vi "写入B版外设配置.vi"(8 "error in (no error)":errorcluster, 10 "外设配置":T1 {"阀型号" items=["垦拓10通阀"]; "总氮x公式0" items=["0", "1"]; "光谱仪类型" items=["1型", "2型", "3型", "2型氙灯联控"]; "泵类型" items=["润泽注射泵", "垦拓注射泵"]}, 11 "MB session in":refnum<class "MB_Master.lvclass">) -> (0 "error out":errorcluster, 3 "MB session out":refnum<class "MB_Master.lvclass">)   [LabVIEW 2016, in "斯坦道总磷总氮.lvlib"]
uses:
  <vilib>/Plasmionique/MB Master/MB_Master/MB_Master.lvclass
  <vilib>/Plasmionique/MB Master/MB_Master_Serial/MB_Master_Serial.lvclass
  C:/Program Files (x86)/National Instruments/LabVIEW 2016/vi.lib/Plasmionique/MB Master/MB_Master/MB_Master.lvclass
  <vilib>/Plasmionique/MB Master/MB Master.lvlib
  <vilib>/Utility/VariantDataType/VariantType.lvlib
panel:
  out "大小":i32
  in  "U32":u32
  in  "SGL":sgl
  in  "U16":u16
  in  "U8":u8
  in  "VISA Resource":refnum<visa-resource-name>
  in  "引用选择":enum16{"MB引用", "自建引用"}(ring)
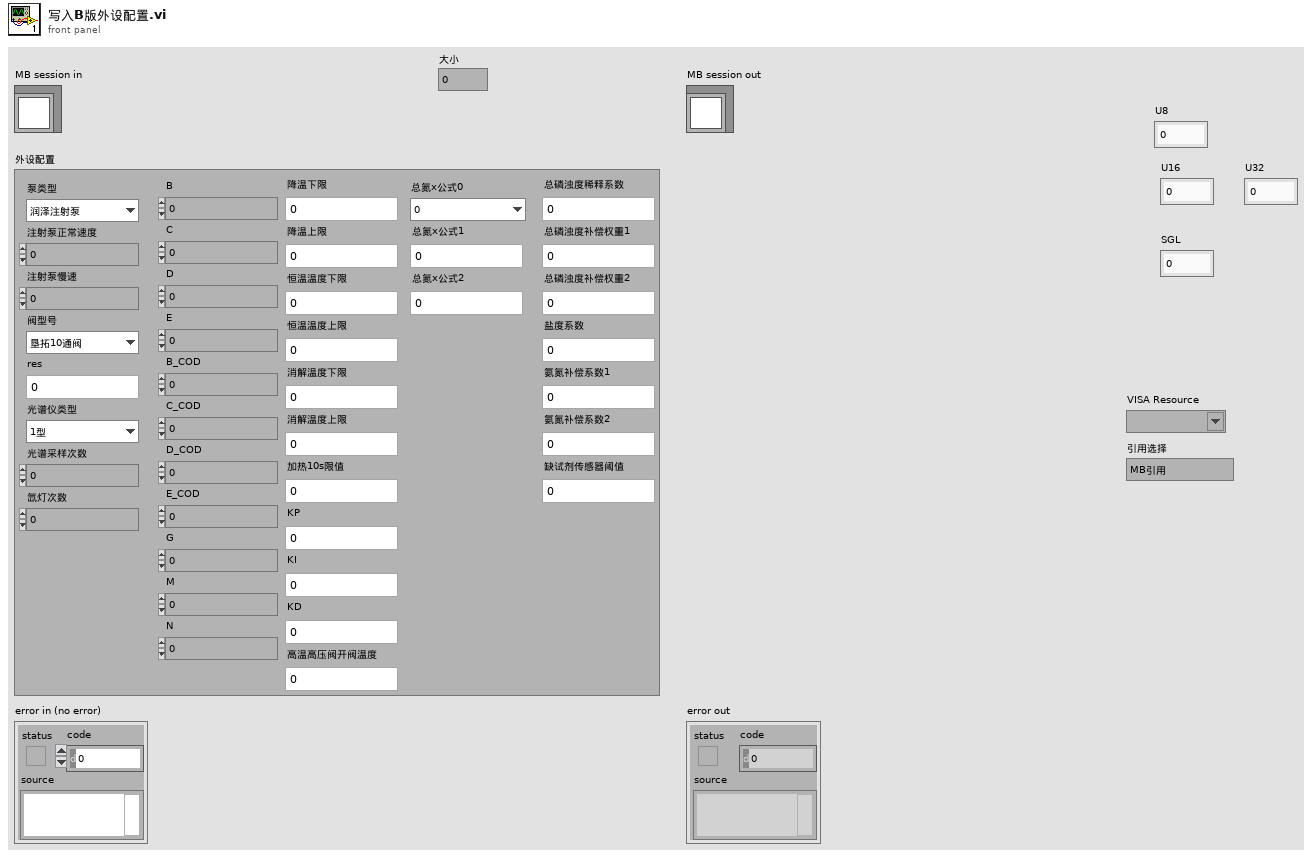
[diagram p1: front panel]
types:
  T1 = typedef "斯坦道总磷总氮.lvlib/V3 B版外设参数.ctl" = cluster{"泵类型":u8, "注射泵正常速度":u32, "注射泵慢速":u32, "阀型号":u8, "res":u8, "光谱仪类型":u8, "光谱采样次数":u8, "氙灯次数":u8, "B":u16, "C":u16, "D":u16, "E":u16, "B_COD":u16, "C_COD":u16, "D_COD":u16, "E_COD":u16, "G":u16, "M":u16, "N":u16, "降温下限":sgl, "降温上限":sgl, "恒温温度下限":sgl, "恒温温度上限":sgl, "消解温度下限":sgl, "消解温度上限":sgl, "加热10s限值":sgl, "KP":sgl, "KI":sgl, "KD":sgl, "高温高压阀开阀温度":sgl, "总氮x公式0":u8, "总氮x公式1":sgl, "总氮x公式2":sgl, "总磷浊度稀释系数":sgl, "总磷浊度补偿权重1":sgl, "总磷浊度补偿权重2":sgl, "盐度系数":sgl, "氨氮补偿系数1":sgl, "氨氮补偿系数2":sgl, "缺试剂传感器阈值":u16}
  T2 = typedef "VariantType.lvlib/Type.ctl" = enum8{"Invalid Type", "Void", "I8", "I16", "I32", "I64", "U8", "U16", "U32", "U64", "Single Float", "Double Float", "Extended Float", "Single Complex", "Double Complex", "Extended Complex", "Enum U8", "Enum U16", "Enum U32", "Enum U64", "Single Float With Unit", "Double Float With Unit", "Extended Float With Unit", "Single Complex with Unit", "Double Complex with Unit", "Extended Complex with Unit", "Boolean", "String", "Path", "Picture", "Tag", "Array", "Cluster", "Variant", "LV Variant", "Waveform", "Timestamp", "Digital Waveform", "Digital Data", "ExpressData", "Refnum", "External Data", "VI", "Poly VI", "LabVIEW Class Instance", "Fixed Point"}
  T3 = cluster{"baud rate (bps)":u32, "stop bits":u16, "parity":u16, "flow control":u16, "timeout":u32, "retries":i32}
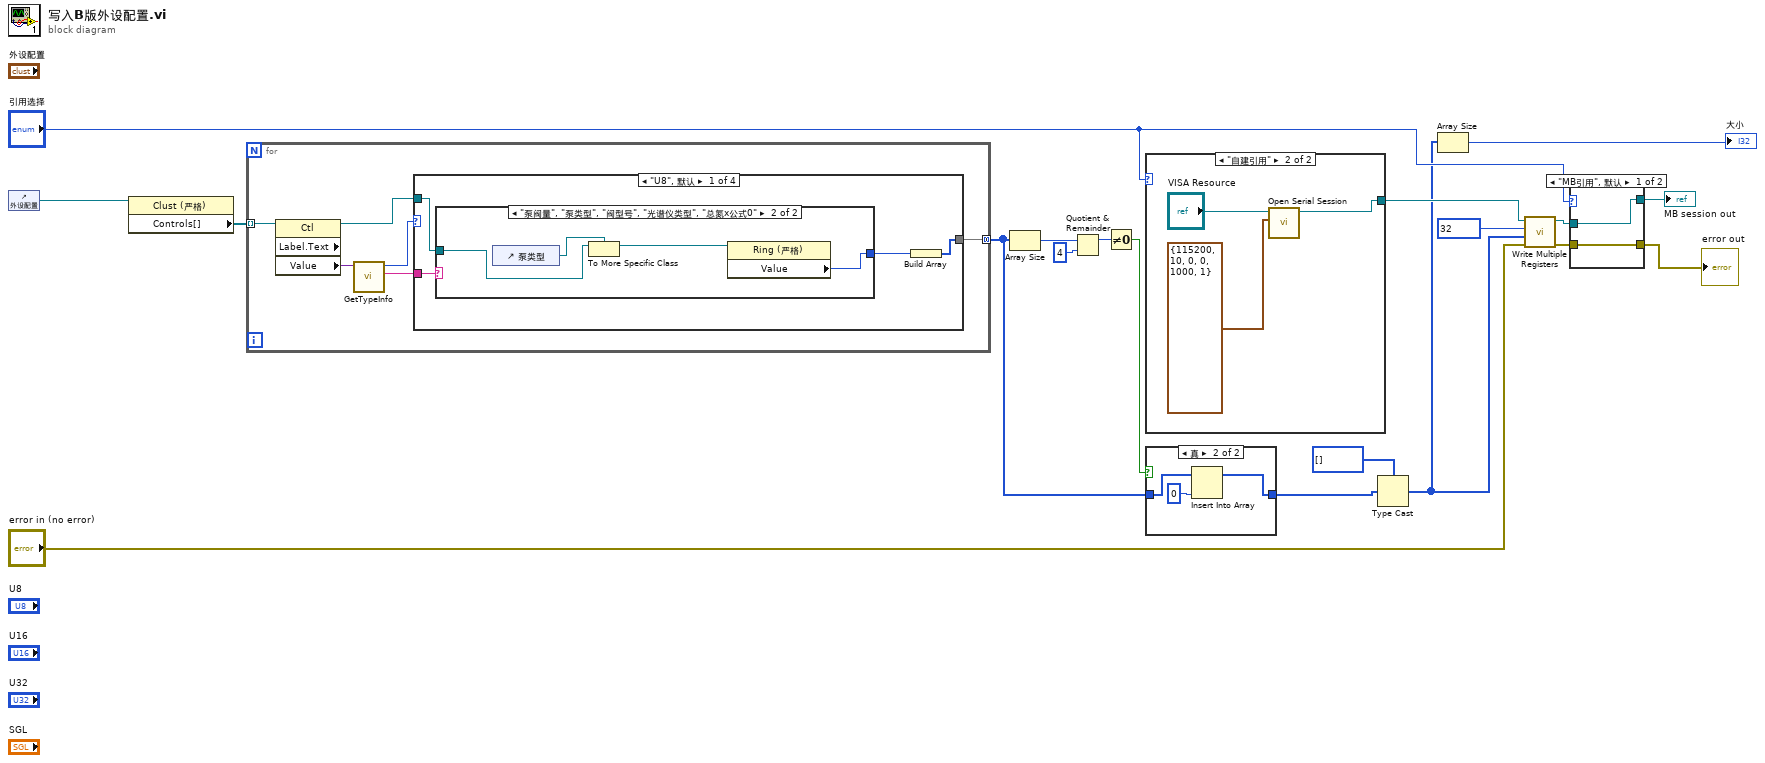
[diagram p0: block diagram]
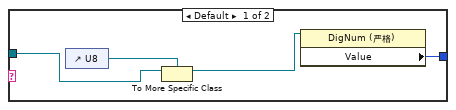
[diagram p3: hidden frame]
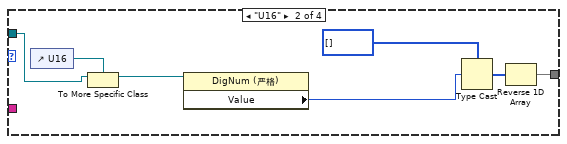
[diagram p4: hidden frame]
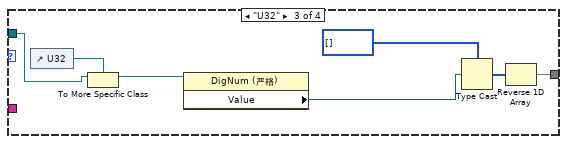
[diagram p5: hidden frame]
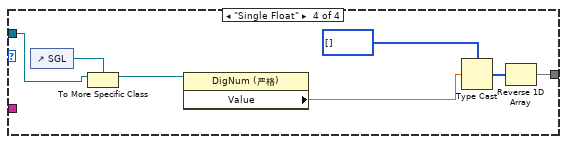
[diagram p6: hidden frame]
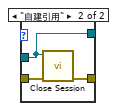
[diagram p7: hidden frame]
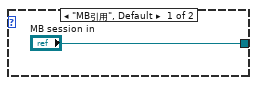
[diagram p8: hidden frame]
diagram:
  n1 = control-ref of="外设配置"() -> (w9:refnum<vi>)
  n2 = property class="Clust (严格)"(reference=w9) -> ("Controls[]"=w11:refnum<vi>[])  [unwired: 1 in, 2 out]
  n3 = for {
    tunnel: w11 -> [w25] mode=indexing
    tunnel: [w21] -> w2 mode=concatenating
    n4 = property class="Ctl" props=["Label", "Text", "Value"](reference=w25) -> (reference out=w22:refnum<vi>, "Value"=w24:variant)  [unwired: 1 in, 2 out]
    n5 = call <vilib>:"GetTypeInfo.vi"("Variant"=w24) -> ("Name"=w20:string, "Type Enum"=w23:T2)  [unwired: 6 in, 3 out]
    n6 = case shown="\"U8\", 默认" w23 {
      tunnel: w22 -> [w27 w44 w51 w58]
      tunnel: [w29 w38 w45 w52] -> w21
      tunnel: w20 -> [w28 _ _ _]
      frame "U8", Default {
        n7 = case shown="\"泵阀量\", \"泵类型\", \"阀型号\", \"光谱仪类型\", \"总氮x公式0\"" w28 {
          tunnel: w27 -> [w32 w37]
          tunnel: [w30 w34] -> w26
          frame Default {
            n8 = control-ref of="U8"() -> (w33:refnum<vi>)
            n9 = To More Specific Class(target class=w33, reference=w32) -> (specific class reference=w31:refnum<vi>)  [unwired: 1 in, 1 out]
            n10 = property class="DigNum (严格)"(reference=w31) -> ("Value"=w30:u8)  [unwired: 1 in, 2 out]
          }
          frame "泵阀量", "泵类型", "阀型号", "光谱仪类型", "总氮x公式0" {
            n11 = control-ref of="泵类型"() -> (w36:refnum<vi>)
            n12 = To More Specific Class(target class=w36, reference=w37) -> (specific class reference=w35:refnum<vi>)  [unwired: 1 in, 1 out]
            n13 = property class="Ring (严格)"(reference=w35) -> ("Value"=w34:u8)  [unwired: 1 in, 2 out]
          }
        }
        n14 = Build Array(w26) -> (w29:u8[])
      }
      frame "U16" {
        n15 = control-ref of="U16"() -> (w43:refnum<vi>)
        n16 = To More Specific Class(target class=w43, reference=w44) -> (specific class reference=w42:refnum<vi>)  [unwired: 1 in, 1 out]
        n17 = property class="DigNum (严格)"(reference=w42) -> ("Value"=w39:u16)  [unwired: 1 in, 2 out]
        n18 = Type Cast(type=u8[] [], x=w39) -> (*(type *) &x=w41:u8[])
        n19 = Reverse 1D Array(array=w41) -> (reversed array=w38:u8[])
      }
      frame "U32" {
        n20 = control-ref of="U32"() -> (w50:refnum<vi>)
        n21 = To More Specific Class(target class=w50, reference=w51) -> (specific class reference=w49:refnum<vi>)  [unwired: 1 in, 1 out]
        n22 = property class="DigNum (严格)"(reference=w49) -> ("Value"=w46:u32)  [unwired: 1 in, 2 out]
        n23 = Type Cast(type=u8[] [], x=w46) -> (*(type *) &x=w48:u8[])
        n24 = Reverse 1D Array(array=w48) -> (reversed array=w45:u8[])
      }
      frame "Single Float" {
        n25 = control-ref of="SGL"() -> (w57:refnum<vi>)
        n26 = To More Specific Class(target class=w57, reference=w58) -> (specific class reference=w56:refnum<vi>)  [unwired: 1 in, 1 out]
        n27 = property class="DigNum (严格)"(reference=w56) -> ("Value"=w53:sgl)  [unwired: 1 in, 2 out]
        n28 = Type Cast(type=u8[] [], x=w53) -> (*(type *) &x=w55:u8[])
        n29 = Reverse 1D Array(array=w55) -> (reversed array=w52:u8[])
      }
    }
  }
  n30 = Array Size(array=w2) -> (size(s)=w5:i32)
  n31 = Quotient & Remainder(x=w5, y=4) -> (x-y*floor(x/y)=w4:i32)  [unwired: 1 out]
  n32 = Not Equal To 0?(x=w4) -> (x != 0?=w3:bool)
  n33 = case shown="\"自建引用\"" "引用选择" {
    tunnel: ["MB session in" w62] -> w17
    frame "MB引用", Default {
    }
    frame "自建引用" {
      n34 = call <vilib>:"Open Serial Session.vi"("Serial Config"=T3 {"baud rate (bps)"=115200, "stop bits"=10, "parity"=0, "flow control"=0, "timeout"=1000, "retries"=1}, "VISA Resource"="VISA Resource") -> ("MB_Serial session"=w62:refnum<class "MB_Master_Serial.lvclass">)  [unwired: 8 in, 1 out]
    }
  }
  n35 = case shown="真" w3 {
    tunnel: w2 -> [w63 w66]
    tunnel: [w63 w64] -> w1
    frame False {
    }
    frame True {
      n36 = Insert Into Array(array=w66, new element=u8 0 ("新元素/子数组")) -> (w64:u8[])  [unwired: 1 in]
    }
  }
  n37 = Type Cast(type=u16[] [], x=w1) -> (*(type *) &x=w8:u16[])
  n38 = Array Size(array=w8) -> (size(s)=→"大小":i32)
  n39 = call <vilib>:"Write Multiple Registers.vi"("error in (no error)"="error in (no error)", "values"=w8, "starting address"=u16 32, "MB session in"=w17) -> ("error out"=w14:errorcluster, "MB session out"=w16:refnum<class "MB_Master.lvclass">)  [unwired: 6 in]
  n40 = case shown="\"MB引用\", 默认" "引用选择" {
    tunnel: w16 -> [w67 w69]
    tunnel: w14 -> [w68 w71]
    tunnel: [w68 w70] -> w13
    tunnel: [w67 w69] -> w12
    frame "MB引用", Default {
    }
    frame "自建引用" {
      n41 = call-dynamic "Close Session.vi"("error in (no error)"=w71, "MB session in"=w69) -> ("error out"=w70:errorcluster)  [unwired: 9 in]
    }
  }
  "MB session out" <- w12
  "error out" <- w13
